vi "RT DC Servo.vi"() -> ()   [LabVIEW 2015]
doc: "The myRIO Custom FPGA Project template acquires button data from the onboard button and displays the button value on a Boolean indicator. The SYS.RDY indicator shows the FPGA status."
uses:
  <vilib>/Utility/error.llb/DialogType.ctl
  Control 1.ctl
  <vilib>/FPGAPlugInAG/myRIO-1900/niLvFpga_Open_myRIO-1900.vi
  <vilib>/rvi/interface/common/dynamic/niFpgaDynamicAddResources.vi
  <vilib>/Utility/error.llb/Error Cluster From Error Code.vi
  <vilib>/rvi/errors/niLvFpgaAdjustHostInterfaceError.vi
  <vilib>/FPGAPlugInAG/Dynamic/niLvFpga_Close_Dynamic.vi
  <vilib>/rvi/interface/nirviOpenFPGA/nirviOpenFPGA.xnode
  FPGA Bitfiles/DCServo_FPGATarget_ParallaxStandard_32fO7nCKYa0.lvbitx
  Parallax Standard Servo (FPGA).vi
  <vilib>/rvi/interface/nirviReadWriteControl/nirviReadWriteControl.xnode
  <vilib>/rvi/interface/nirviCloseFPGA/nirviCloseFPGA.xnode
  NiFpgaLv.dll
  <vilib>/rvi/interface/Simulation/niFpgaSimulationCallBeginRW.vi
panel:
  in  "START/STOP":bool
  out "Sudut":dbl(knob) min=0.0 max=180.0 step=1.0 scale=0.0..90.0
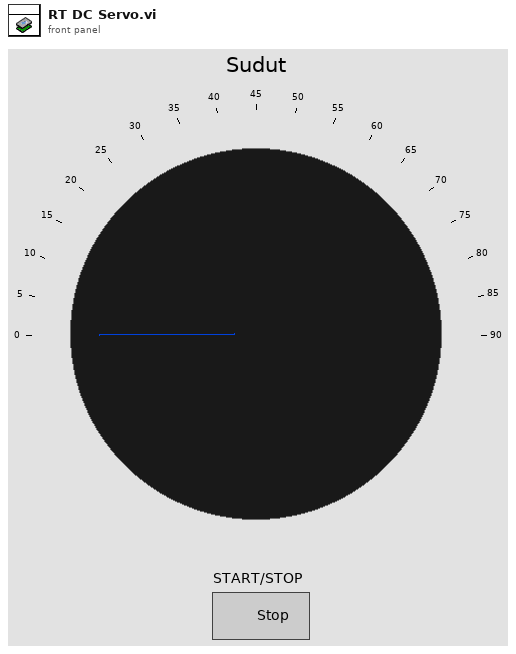
[diagram p1: front panel]
types:
  T1 = typedef "Control 1.ctl" = enum16{"START", "Go to 10", "Delay1 5s", "Go to 45", "Delay2 5s", "Go to 60", "Delay3 5s", "Go to 90", "Delay4 5s", "Go to 0", "Continued?", "Stop"}
  T2 = typedef "DialogType.ctl" = u16
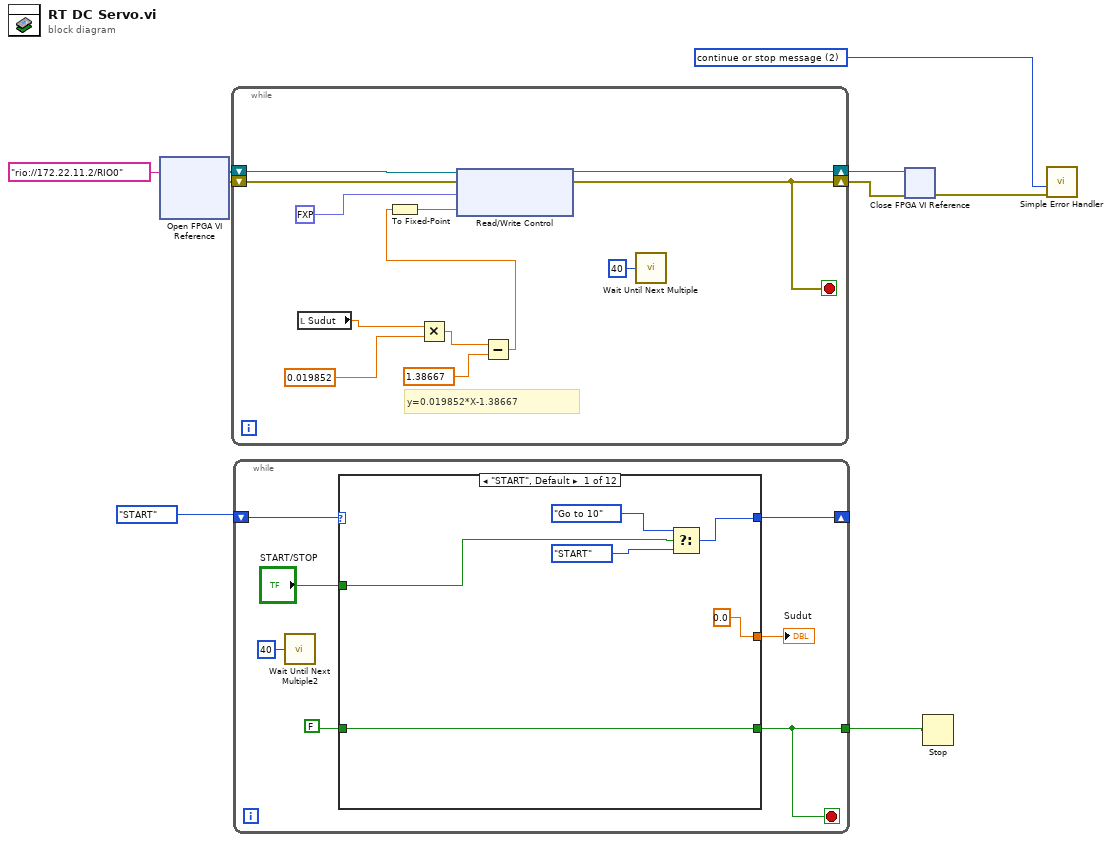
[diagram p0: block diagram]
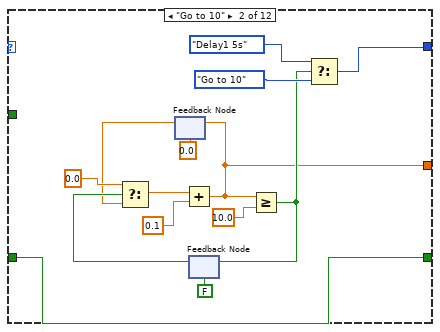
[diagram p2: hidden frame]
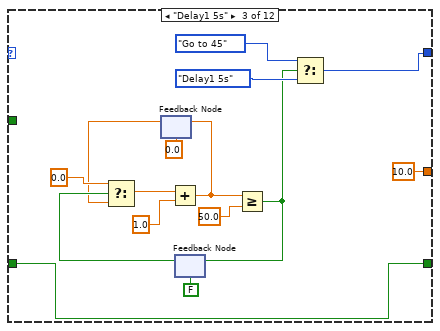
[diagram p3: hidden frame]
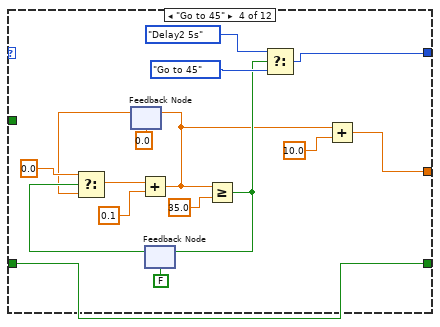
[diagram p4: hidden frame]
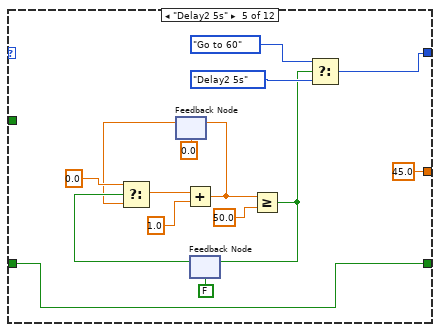
[diagram p5: hidden frame]
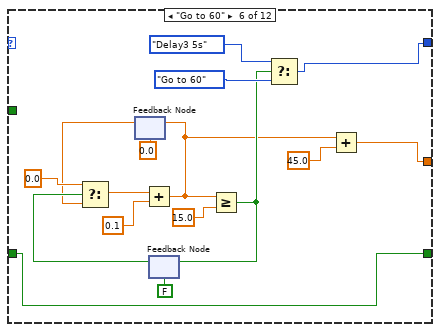
[diagram p6: hidden frame]
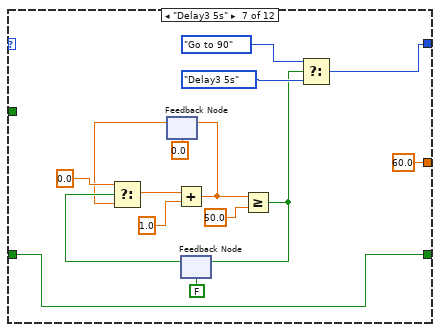
[diagram p7: hidden frame]
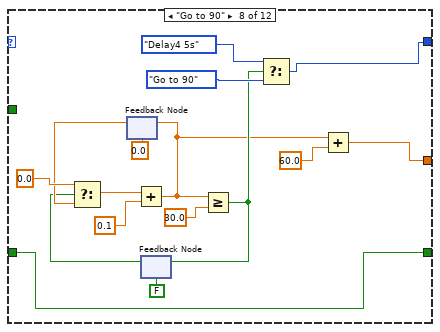
[diagram p8: hidden frame]
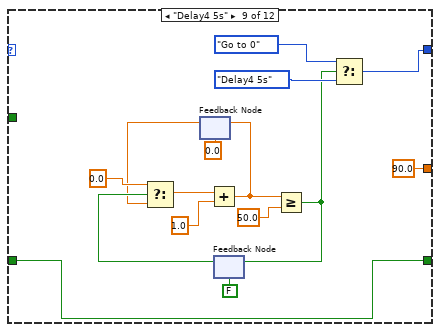
[diagram p9: hidden frame]
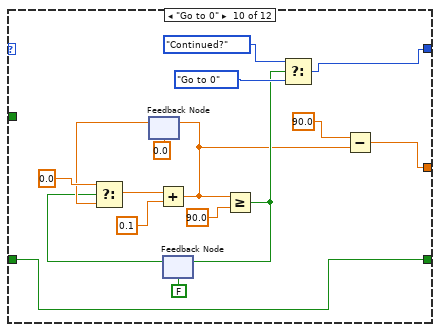
[diagram p10: hidden frame]
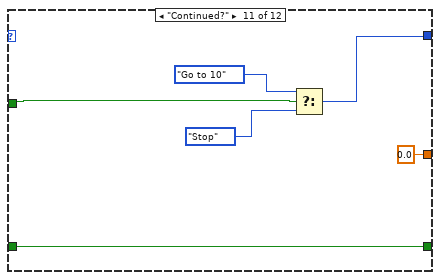
[diagram p11: hidden frame]
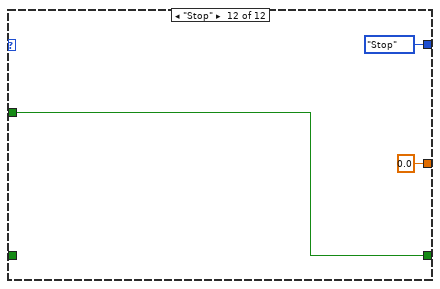
[diagram p12: hidden frame]
diagram:
  w3 = T2 2 items=["no dialog", "OK message", "continue or stop message", "OK message + warnings", "continue/stop + warnings"] ("type of dialog (OK msg:1)")
  n1 = xnode "Open FPGA VI Reference"("resource name"=tag "rio://172.22.11.2/RIO0") -> ("FPGA VI Reference Out"=w8:refnum<k20>, "error out"=w7:errorcluster)  [unwired: 1 in]
  n2 = while {
    shift-right: [w18] -> w6
    shift-left: w8 -> [w21]
    shift-right: [w17] -> w5
    shift-left: w7 -> [w20]
    stop <- w17 stop-if-true
    # "y=0.019852*X-1.38667"
    n3 = local read "Sudut"() -> (w10:dbl)
    n4 = Multiply(x=w10, y=0.019852) -> (x*y=w14:dbl)
    n5 = Subtract(x=w14, y=1.38667) -> (x-y=w11:dbl)
    n6 = To Fixed-Point(number=w11) -> (fixed-point=w12:fxp<+/-,32,16>)  [unwired: 1 in]
    n7 = xnode "Read/Write Control"("FPGA VI Reference In"=w21, "error in"=w20, "servo_0_ccw offset"=fxp<+/-,32,4> 0.0, "servo_0_ccw angle"=w12) -> ("FPGA VI Reference Out"=w18:refnum<k20>, "error out"=w17:errorcluster)
    n8 = call "Wait Until Next Multiple"("Count(mSec)"=u32 40) -> ()  [unwired: 1 out]
  }
  n9 = while {
    shift-right: [w27] -> _
    shift-left: Control_1."START" -> [w28]
    tunnel: [w23] -> w1
    stop <- w23 stop-if-true
    n10 = call "Wait Until Next Multiple2"("Count(mSec)"=u32 40) -> ()  [unwired: 1 out]
    n11 = case shown="\"START\", Default" w28 {
      tunnel: [w33 w47 w51 w69 w82 w98 w113 w130 w144 w161 w176 Control_1."Stop" ("f")] -> w27
      tunnel: [0.0 w36 10.0 w66 45.0 w97 60.0 w129 90.0 w160 0.0 0.0] -> w26
      tunnel: "START/STOP" -> [w30 _ _ _ _ _ _ _ _ _ w174 w180]
      tunnel: [w29 w35 w49 w64 w80 w95 w111 w126 w142 w157 w173 w180] -> w23
      tunnel: FALSE -> [w29 w35 w49 w64 w80 w95 w111 w126 w142 w157 w173 _]
      frame "START", Default {
        n12 = Select(t=Control_1."Go to 10", s=w30, f=Control_1."START") -> (s? t:f=w33:T1)
      }
      frame "Go to 10" {
        n13 = feedback #1(0.0) -> (w38:dbl)
        n14 = feedback #2(FALSE) -> (w40:bool)
        n15 = Select(t=0.0, s=w40, f=w38) -> (s? t:f=w42:dbl)
        n16 = Add(x=w42, y=0.1) -> (x+y=w36:dbl)
        n17 = feedback-in #1(w36) -> ()
        n18 = Greater Or Equal?(x=w36, y=10.0) -> (x >= y?=w41:bool)
        n19 = feedback-in #2(w41) -> ()
        n20 = Select(t=Control_1."Delay1 5s", s=w41, f=Control_1."Go to 10") -> (s? t:f=w47:T1)
      }
      frame "Delay1 5s" {
        n21 = feedback #3(0.0) -> (w53:dbl)
        n22 = feedback #4(FALSE) -> (w56:bool)
        n23 = Select(t=0.0, s=w56, f=w53) -> (s? t:f=w58:dbl)
        n24 = Add(x=w58, y=1.0) -> (x+y=w54:dbl)
        n25 = feedback-in #3(w54) -> ()
        n26 = Greater Or Equal?(x=w54, y=50.0) -> (x >= y?=w57:bool)
        n27 = feedback-in #4(w57) -> ()
        n28 = Select(t=Control_1."Go to 45", s=w57, f=Control_1."Delay1 5s") -> (s? t:f=w51:T1)
      }
      frame "Go to 45" {
        n29 = feedback #5(0.0) -> (w71:dbl)
        n30 = feedback #6(FALSE) -> (w73:bool)
        n31 = Select(t=0.0, s=w73, f=w71) -> (s? t:f=w68:dbl)
        n32 = Add(x=w68, y=0.1) -> (x+y=w65:dbl)
        n33 = feedback-in #5(w65) -> ()
        n34 = Greater Or Equal?(x=w65, y=35.0) -> (x >= y?=w74:bool)
        n35 = feedback-in #6(w74) -> ()
        n36 = Select(t=Control_1."Delay2 5s", s=w74, f=Control_1."Go to 45") -> (s? t:f=w69:T1)
        n37 = Add(x=w65, y=10.0) -> (x+y=w66:dbl)
      }
      frame "Delay2 5s" {
        n38 = feedback #7(0.0) -> (w84:dbl)
        n39 = feedback #8(FALSE) -> (w87:bool)
        n40 = Select(t=0.0, s=w87, f=w84) -> (s? t:f=w89:dbl)
        n41 = Add(x=w89, y=1.0) -> (x+y=w85:dbl)
        n42 = feedback-in #7(w85) -> ()
        n43 = Greater Or Equal?(x=w85, y=50.0) -> (x >= y?=w88:bool)
        n44 = feedback-in #8(w88) -> ()
        n45 = Select(t=Control_1."Go to 60", s=w88, f=Control_1."Delay2 5s") -> (s? t:f=w82:T1)
      }
      frame "Go to 60" {
        n46 = feedback #9(0.0) -> (w102:dbl)
        n47 = feedback #10(FALSE) -> (w104:bool)
        n48 = Select(t=0.0, s=w104, f=w102) -> (s? t:f=w100:dbl)
        n49 = Add(x=w100, y=0.1) -> (x+y=w96:dbl)
        n50 = feedback-in #9(w96) -> ()
        n51 = Greater Or Equal?(x=w96, y=15.0) -> (x >= y?=w105:bool)
        n52 = feedback-in #10(w105) -> ()
        n53 = Select(t=Control_1."Delay3 5s", s=w105, f=Control_1."Go to 60") -> (s? t:f=w98:T1)
        n54 = Add(x=w96, y=45.0) -> (x+y=w97:dbl)
      }
      frame "Delay3 5s" {
        n55 = feedback #11(0.0) -> (w115:dbl)
        n56 = feedback #12(FALSE) -> (w118:bool)
        n57 = Select(t=0.0, s=w118, f=w115) -> (s? t:f=w120:dbl)
        n58 = Add(x=w120, y=1.0) -> (x+y=w116:dbl)
        n59 = feedback-in #11(w116) -> ()
        n60 = Greater Or Equal?(x=w116, y=50.0) -> (x >= y?=w119:bool)
        n61 = feedback-in #12(w119) -> ()
        n62 = Select(t=Control_1."Go to 90", s=w119, f=Control_1."Delay3 5s") -> (s? t:f=w113:T1)
      }
      frame "Go to 90" {
        n63 = feedback #13(0.0) -> (w134:dbl)
        n64 = feedback #14(FALSE) -> (w128:bool)
        n65 = Select(t=0.0, s=w128, f=w134) -> (s? t:f=w132:dbl)
        n66 = Add(x=w132, y=0.1) -> (x+y=w127:dbl)
        n67 = feedback-in #13(w127) -> ()
        n68 = Greater Or Equal?(x=w127, y=30.0) -> (x >= y?=w136:bool)
        n69 = feedback-in #14(w136) -> ()
        n70 = Select(t=Control_1."Delay4 5s", s=w136, f=Control_1."Go to 90") -> (s? t:f=w130:T1)
        n71 = Add(x=w127, y=60.0) -> (x+y=w129:dbl)
      }
      frame "Delay4 5s" {
        n72 = feedback #15(0.0) -> (w146:dbl)
        n73 = feedback #16(FALSE) -> (w149:bool)
        n74 = Select(t=0.0, s=w149, f=w146) -> (s? t:f=w151:dbl)
        n75 = Add(x=w151, y=1.0) -> (x+y=w147:dbl)
        n76 = feedback-in #15(w147) -> ()
        n77 = Greater Or Equal?(x=w147, y=50.0) -> (x >= y?=w150:bool)
        n78 = feedback-in #16(w150) -> ()
        n79 = Select(t=Control_1."Go to 0", s=w150, f=Control_1."Delay4 5s") -> (s? t:f=w144:T1)
      }
      frame "Go to 0" {
        n80 = feedback #17(0.0) -> (w165:dbl)
        n81 = feedback #18(FALSE) -> (w162:bool)
        n82 = Select(t=0.0, s=w162, f=w165) -> (s? t:f=w163:dbl)
        n83 = Add(x=w163, y=0.1) -> (x+y=w158:dbl)
        n84 = feedback-in #17(w158) -> ()
        n85 = Greater Or Equal?(x=w158, y=90.0) -> (x >= y?=w167:bool)
        n86 = feedback-in #18(w167) -> ()
        n87 = Select(t=Control_1."Continued?", s=w167, f=Control_1."Go to 0") -> (s? t:f=w161:T1)
        n88 = Subtract(x=90.0 ("y"), y=w158) -> (x-y=w160:dbl)
      }
      frame "Continued?" {
        n89 = Select(t=Control_1."Go to 10", s=w174, f=Control_1."Stop") -> (s? t:f=w176:T1)
      }
      frame "Stop" {
      }
    }
    "Sudut" <- w26
  }
  n90 = xnode "Close FPGA VI Reference"("FPGA VI Reference In"=w6, "error in"=w5) -> ("error out"=w4:errorcluster)
  n91 = Stop(stop? (T)=w1) -> ()
  n92 = call <vilib>:"Simple Error Handler.vi"("type of dialog (OK msg:1)"=w3, "error in (no error)"=w4) -> ()  [unwired: 3 in, 5 out]
